vi "PulserGlobals.vi"() -> ()   [LabVIEW 2022 SP3]
uses:
  pulser.ctl
  Daxsonics/-DaxSubroutines/Daxsonics_Pulsers.ctl
  JSR/Controls/JSR Complete.ctl
  JSR/Controls/JSR Pulse.ctl
  JSR/Controls/Damping.ctl
  JSR/Controls/Energy.ctl
  JSR/Controls/Z.ctl
  JSR/Controls/Volt.ctl
  JSR/Controls/JSR Recieve.ctl
  JSR/Controls/Mode.ctl
  JSR/Controls/HPF.ctl
  JSR/Controls/LPF.ctl
  JSR/Controls/Gain.ctl
  JSR/Controls/JSR Trigger.ctl
  JSR/Controls/Trig Limit.ctl
  JSR/Controls/Trig Source.ctl
  JSR/Controls/PRF.ctl
  UTEX/Controls/UTEX Controls.ctl
panel:
  in  "UT340 Controls":T1={"High Pass On"=FALSE, "High Pass Filter (MHz)"=1, "Low Pass On"=FALSE, "Low Pass Filter (MHz)"=20, "PE Gain (dB)"=1, "Voltage"=100, "Pulse Width (ns)"=2.0, "Mode"=FALSE, "PC Gain (dB)"=1, "Trig Source"=FALSE, "Rep Rate (Hz)"=0, "PULSE"=FALSE} {"Low Pass Filter (MHz)" min=20 step=1; "High Pass Filter (MHz)" min=1 max=20 step=1; "Pulse Width (ns)" min=2.0 max=71.75; "Voltage" min=100 max=250 step=2; "PC Gain (dB)" min=-6 max=60 step=1; "PE Gain (dB)" min=-6 max=60 step=1}
  in  "UTEX VISA":refnum<visa-resource-name>="COM4"
  in  "JSR Settings":T2={"JSR Pulse Settings"={"Damping"=59, "Pulse Energy Level"=2, "Pulser Impedance"=0, "Pulser Voltage (V)"=100}, "JSR Receive Settings"={"Receiver Mode"=0, "High Pass Filter"=5000, "Low Pass Filter"=50, "Gain (dB)"=50}, "JSR Trigger Settings"={"External Trigger Limit"=0, "Trigger Source"=1, "PRF (Hz)"=1.75}} {"JSR Trigger Settings"."PRF (Hz)" items=["100 Hz"=0.1, "200 Hz"=0.2, "400 Hz"=0.4, "600 Hz"=0.6, "800 Hz"=0.8, "1000 Hz"=1.0, "1250 Hz"=1.25, "1500 Hz"=1.5, "1750 Hz"=1.75, "2000 Hz"=2.0, "2500 Hz"=2.5, "3000 Hz"=3.0, "3500 Hz"=3.5, "4000 Hz"=4.0, "4500 Hz"=4.5, "5000 Hz"=5.0]; "JSR Trigger Settings"."Trigger Source" items=["Internal", "External"]; "JSR Trigger Settings"."External Trigger Limit" items=["No Limit", "5 kHz"]; "JSR Receive Settings"."Gain (dB)" min=-13 max=66 step=1; "JSR Receive Settings"."Low Pass Filter" items=["5 MHz"=5, "10 MHz"=10, "15 MHz"=15, "22.5 MHz"=22, "35 MHz"=35, "50 MHz"=50]; "JSR Receive Settings"."High Pass Filter" items=["DC"=0, "1 MHz"=1000, "2.5 MHz"=2500, "5 MHz"=5000, "7.5 MHz"=7500, "12.5 MHz"=12500]; "JSR Receive Settings"."Receiver Mode" items=["Echo", "Through"]; "JSR Pulse Settings"."Pulser Voltage (V)" items=["100"=100, "125"=125, "150"=150, "175"=175, "200"=200, "225"=225, "250"=250, "275"=275, "300"=300, "325"=325, "350"=350, "375"=375, "400"=400, "425"=425, "450"=450, "475"=475]; "JSR Pulse Settings"."Pulser Impedance" items=["High z", "Low z"]; "JSR Pulse Settings"."Pulse Energy Level" items=["0 (Minimum)", "1", "2", "3 (Maximum)"]; "JSR Pulse Settings"."Damping" items=["331 Ohms"=331, "198 Ohms"=198, "142 Ohms"=142, "110 Ohms"=110, "92 Ohms"=92, "77 Ohms"=77, "67 Ohms"=67, "59 Ohms"=59, "52 Ohms"=52, "47 Ohms"=47, "43 Ohms"=43, "39 Ohms"=39, "37 Ohms"=37, "34 Ohms"=34, "32 Ohms"=32, "30 Ohms"=30]}
  in  "JSR VISA":refnum<visa-resource-name>="COM8"
  in  "Daxsonics Name":T17
  in  "Panametrics":refnum<visa-resource-name>="GPIB1::1::INSTR"
  in  "Agilent":refnum<visa-resource-name>="GPIB::10"
  in  "Divide prf by":i32=2
  in  "Tabor":string="ASRL3::INSTR"
  in  "prf (kHz)":dbl=1.0 format="%.3f"
  in  "Therapy Settings":T18 {"Time (s)" format="%.2e"; "Therapy Delay (ms)" format="%.2f"; "time therapy on (s)" format="%.2f"; "Therapy amplitude (mV)" format="%.2f"; "Therapy frequency (MHz)" format="%.3f"}
  in  "Pulser Gain (Single)":sgl format="%.1f"
  in  "Pulser Gain":sgl[](array[numeric]) format="%.1f"
  in  "Daxsonics VISA":refnum<visa-resource-name>="COM8"
  in  "Contrast Excitation":u16(ring) items=["Tone Burst", "Chirp"]
  out "Pan Scan Settings":T19
  in  "Freq. [MHz]":i16=40
  in  "Voltage [V]":i16=35
  in  "Pulse mode":u16(ring)=3 caption="Puls mode" items=["Half cycle positive", "Half cycle negative", "Full cycle positive", "Full cycle negative"]
  in  "Pulser":T20
  # "Ron's pulser"
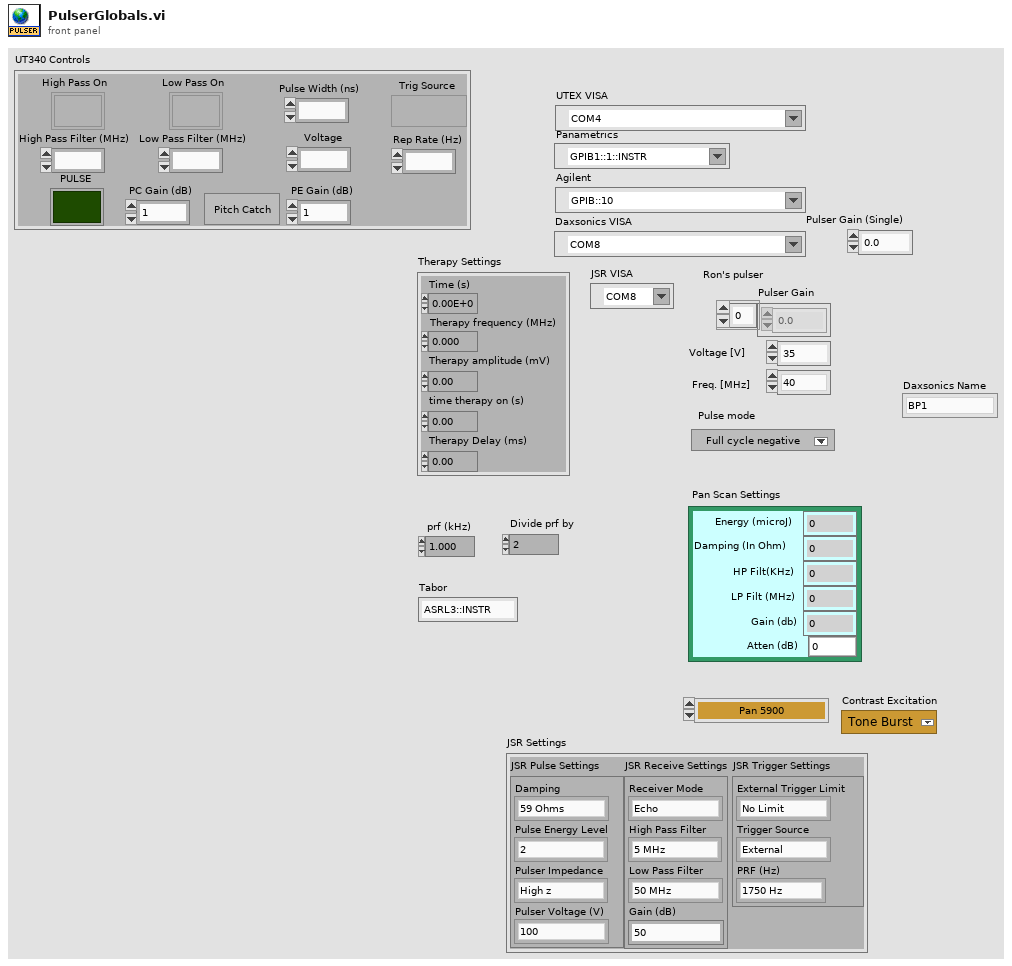
[diagram p1: front panel]
types:
  T1 = typedef "UTEX Controls.ctl" = cluster{"High Pass On":bool, "High Pass Filter (MHz)":i16, "Low Pass On":bool, "Low Pass Filter (MHz)":i16, "PE Gain (dB)":i16, "Voltage":i16, "Pulse Width (ns)":dbl, "Mode":bool, "PC Gain (dB)":i16, "Trig Source":bool, "Rep Rate (Hz)":i16, "PULSE":bool}
  T2 = typedef "JSR Complete.ctl" = cluster{"JSR Pulse Settings":T3, "JSR Receive Settings":T8, "JSR Trigger Settings":T13}
  T3 = typedef "JSR Pulse.ctl" = cluster{"Damping":T4, "Pulse Energy Level":T5, "Pulser Impedance":T6, "Pulser Voltage (V)":T7}
  T4 = typedef "Damping.ctl" = i16
  T5 = typedef "Energy.ctl" = u16
  T6 = typedef "Z.ctl" = u16
  T7 = typedef "Volt.ctl" = i16
  T8 = typedef "JSR Recieve.ctl" = cluster{"Receiver Mode":T9, "High Pass Filter":T10, "Low Pass Filter":T11, "Gain (dB)":T12}
  T9 = typedef "Mode.ctl" = i8
  T10 = typedef "HPF.ctl" = u16
  T11 = typedef "LPF.ctl" = u16
  T12 = typedef "Gain.ctl" = i8
  T13 = typedef "JSR Trigger.ctl" = cluster{"External Trigger Limit":T14, "Trigger Source":T15, "PRF (Hz)":T16}
  T14 = typedef "Trig Limit.ctl" = i8
  T15 = typedef "Trig Source.ctl" = i8
  T16 = typedef "PRF.ctl" = dbl
  T17 = typedef "Daxsonics_Pulsers.ctl" = enum16{"BP1", "BP2_A", "BP2_B", "10ERS8", "New2021"}
  T18 = cluster{"Therapy frequency (MHz)":dbl, "Therapy amplitude (mV)":dbl, "time therapy on (s)":dbl, "Therapy Delay (ms) ":dbl, "Time (s)":dbl}
  T19 = cluster{"Energy (microJ)":u8, "Damping (In Ohm)":u8, "HP Filt(KHz) ":u16, "LP Filt (MHz)":u8, "Gain (db)":u8, "Atten (dB)":sgl}
  T20 = typedef "pulser.ctl" = enum16{"Pan 5900", "Daxsonics", "Agilent 33xxx", "UTEX", "JSR", "WMC Mono-Cycle", "No Pulser", "NYU AVTECH", "Tabor W1281A", "Pan 5800", "Unlisted", "Tabor WX2182B"}
diagram:
